vi "Set And_Save_Channel_Map.vi"(2 "error in":errorcluster, 3 "Filename (.ini)":string="channels_map_default.ini") -> (0 "error out":errorcluster, 1 "Channels map":T1[](array[typedef]))   [LabVIEW 2021]
uses:
  Channel_Cluster.ctl
  Channel_Map_Global.vi
  <vilib>/Utility/config.llb/Write Key (U32).vi
  <vilib>/Utility/config.llb/NI_LVConfig.lvlib
panel:
  # "Remember that config files are .ini, \nconfig file will be save in ...\\Config_Files\\(filename).ini"
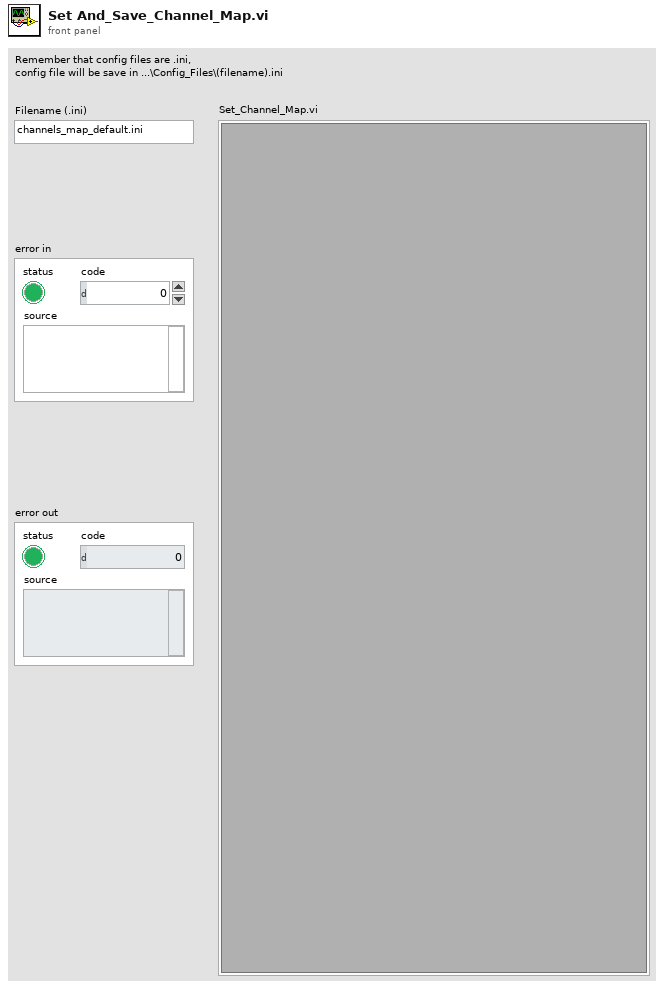
[diagram p1: front panel]
types:
  T1 = typedef "Channel_Cluster.ctl" = cluster{"Channel name":string, "Channel":u8}
  T2 = typedef "NI_LVConfig.lvlib/Config Data RefNum.ctl" = refnum<k1>
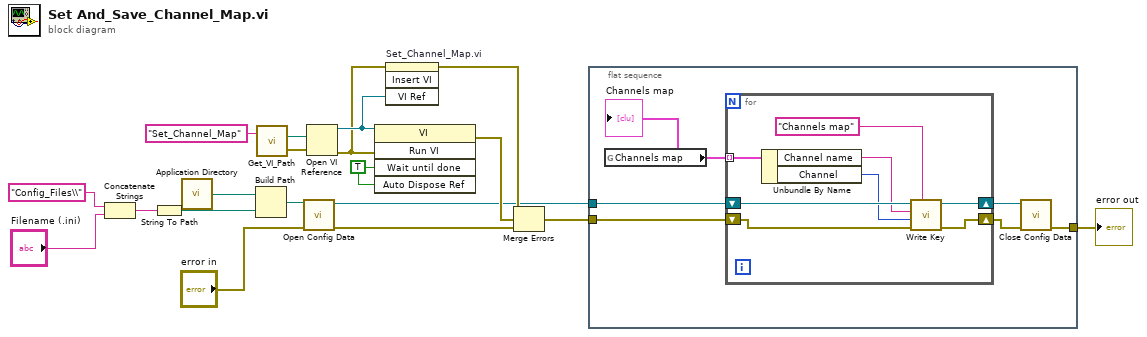
[diagram p0: block diagram]
diagram:
  w13 = TRUE ("Wait Until Done")
  n1 = Concatenate Strings("Config_Files\\" ("string"), "Filename (.ini)") -> (w2:string)
  n2 = String To Path(string=w2) -> (path=w10:path)
  n3 = call <vilib>:"Application Directory.vi"() -> ("Application Directory"=w19:path)
  n4 = Build Path(base path=w19, name or relative path=w10) -> (appended path=w18:path)
  n5 = call "Get_VI_Path.vi"("VI name (no .vi)"="Set_Channel_Map") -> ("error out"=w14:errorcluster, "File Path"=w16:path)  [unwired: 1 in]
  n6 = call <vilib>:"Open Config Data.vi"("error in (no error)"="error in", "configuration file path"=w18) -> ("error out"=w9:errorcluster, "refnum"=w5:T2)  [unwired: 7 in, 1 out]
  n7 = Open VI Reference(vi path=w16, error in (no error)=w14) -> (vi reference=w12:refnum<vi>, error out=w11:errorcluster)  [unwired: 4 in]
  n8 = invoke class="VI" method="Run VI"(reference=w12, error in=w11, "Wait until done"=w13, "Auto Dispose Ref"=w13) -> (error out=w8:errorcluster)  [unwired: 1 in, 4 out]
  n9 = invoke on="Set_Channel_Map.vi" class="SubPnl" method="Insert VI"(error in=w11, "VI Ref"=w12) -> (error out=w7:errorcluster)  [unwired: 2 in, 3 out]
  n10 = Merge Errors(w7, w8, w9) -> (w6:errorcluster)
  n11 = flat-sequence {
    tunnel: w6 -> [w24]
    tunnel: w5 -> [w23]
    tunnel: [w20] -> w1
    frame #0 {
      n12 = global read "Channel_Map_Global.vi" "Channels map"() -> (w25:T1[])
      "Channels map" <- w25
      n13 = for {
        tunnel: w25 -> [w33] mode=indexing
        shift-right: [w28] -> w21
        shift-left: w24 -> [w26]
        shift-right: [w27] -> w22
        shift-left: w23 -> [w32]
        n14 = Unbundle By Name(w33) -> ("Channel name"=w31:string, "Channel"=w30:u8)
        n15 = call-poly <vilib>:"Write Key.vi"("section"="Channels map", "error in (no error)"=w26, "value"=w30, "key"=w31, "refnum"=w32) -> ("error out"=w28:errorcluster, "refnum out"=w27:T2)  [unwired: 4 in, 1 out]
      }
      n16 = call <vilib>:"Close Config Data.vi"("error in (no error)"=w21, "refnum"=w22) -> ("error out"=w20:errorcluster)  [unwired: 8 in, 1 out]
    }
  }
  "error out" <- w1
